vi "TestExec.Set Position.vi"(7 "Module Q Name":string, 8 "error in":errorcluster, 10 "Position":string, 11 "Q In":refnum<queue>) -> (0 "error out":errorcluster, 3 "Q Out":refnum<queue>)   [LabVIEW 2018]
uses:
  <vilib>/KATE/Queues/Q.Element.ctl
  <vilib>/KATE/Queues/Queue Utils.lvlib
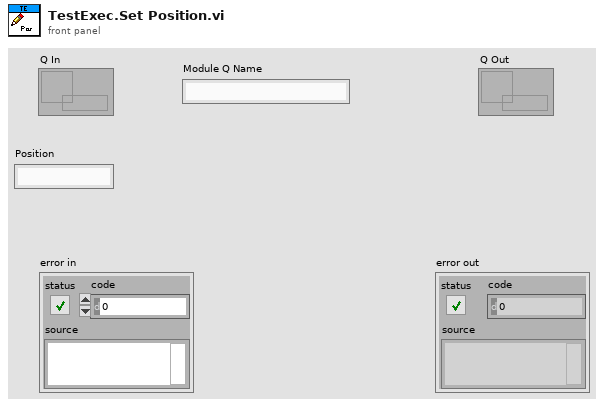
[diagram p1: front panel]
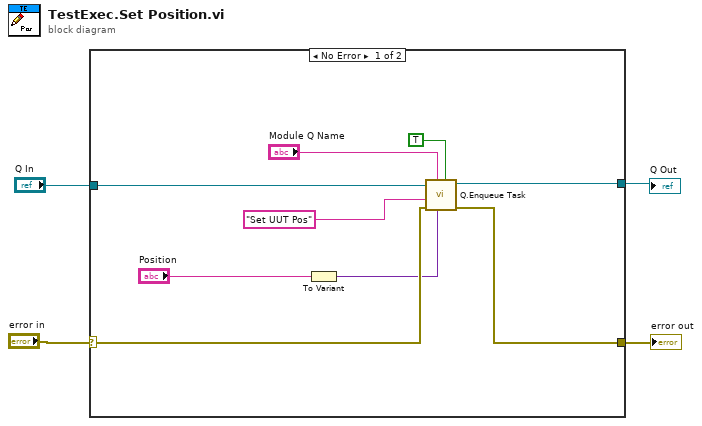
[diagram p0: block diagram]
diagram:
  n1 = case shown="No Error" "error in" {
    selector: "error in" -> [w11 w15]
    tunnel: [w12 w15] -> w3
    tunnel: [w6 w14] -> w2
    tunnel: "Q In" -> [w5 w14]
    frame No Error {
      n2 = To Variant(anything="Position") -> (Variant=w10:variant)
      n3 = call <vilib>:"Q.Enqueue Task.vi"("Top of Q"=TRUE, "Data1"=w10, "Q Name"="Module Q Name", "Error In"=w11, "Task Name"="Set UUT Pos" ("Cmd"), "Q In"=w5) -> ("error out"=w12:errorcluster, "Q Out"=w6:refnum<queue>)  [unwired: 4 in]
    }
    frame Error {
    }
  }
  "error out" <- w3
  "Q Out" <- w2
